vi "close_data_log.vi"(8 "error in (no error)":errorcluster, 11 "pcfs_hdf5_log in":refnum<class "pcfs_hdf5_log.lvclass">) -> (0 "error out":errorcluster, 3 "pcfs_hdf5_log out":refnum<class "pcfs_hdf5_log.lvclass">)   [LabVIEW 2015, in "pcfs_hdf5_log.lvclass"]
uses:
  pcfs_hdf5_log.lvclass
  pcfs_hdf5_log.lvclass/pcfs_hdf5_log.ctl
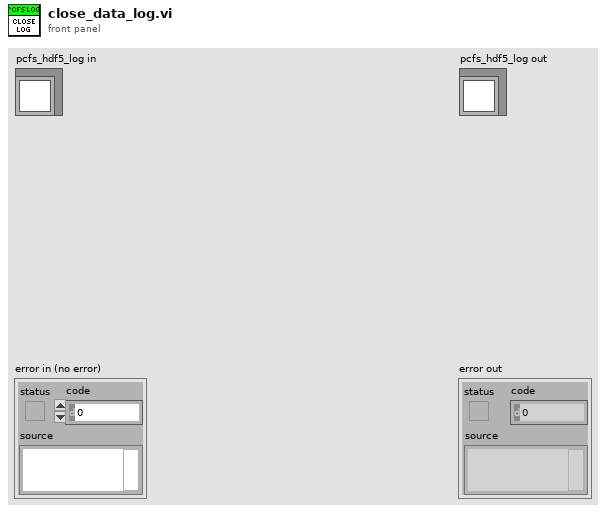
[diagram p1: front panel]
types:
  T1 = typedef "HDF5 Ref.ctl" = refnum<k1>
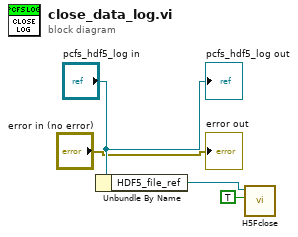
[diagram p0: block diagram]
diagram:
  n1 = Unbundle By Name("pcfs_hdf5_log in") -> ("HDF5_file_ref"=w4:T1)
  n2 = call <vilib>:"H5Fclose.vi"("Close All Open Objects (T)"=TRUE, "HDF5 Ref"=w4) -> ()  [unwired: 7 in, 1 out]
  "error out" <- "error in (no error)"
  "pcfs_hdf5_log out" <- "pcfs_hdf5_log in"
